vi "SubPanelBasicFlow.vi"(0 "VI Reference In":refnum<vi>, 1 "Label (VI Title)":string="Default", 11 "error in (no error)":errorcluster) -> (4 "VI Reference Out":refnum<vi>, 15 "error out":errorcluster)   [LabVIEW 2016, in "Drona Test.lvlib"]
uses:
  Drona Test.lvlib
  main/apis/Stimulus/ValueSignal/ValueSignalByPathString.vi
  main/apis/Assert/AssertControlValue/Equal.vi
  <vilib>/addons/_JKI Toolkits/Caraya/classes/Assert/Assert Not Error.vi
  <vilib>/addons/_JKI Toolkits/Caraya/classes/Test/Test.lvclass
  main/Drona.lvlib
  <vilib>/addons/_JKI Toolkits/Caraya/classes/Assert/Assert.lvclass
  main/apis/Assert/AssertControlValue/AssertControlValue.lvlib
  main/apis/Stimulus/ValueSignal/ValueSignal.lvlib
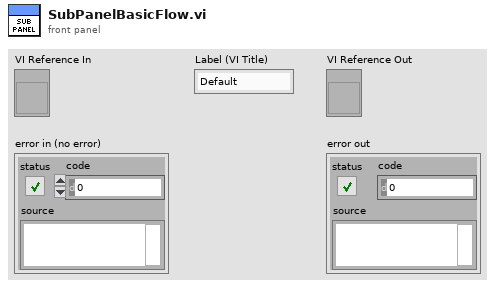
[diagram p1: front panel]
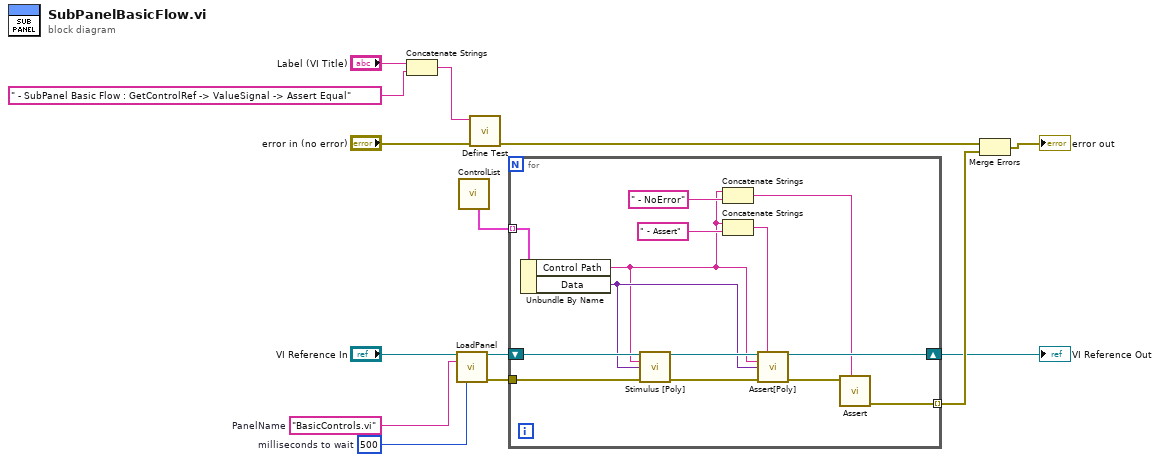
[diagram p0: block diagram]
diagram:
  w4 = u32 500  # milliseconds to wait
  w5 = "BasicControls.vi"  # PanelName
  n1 = Concatenate Strings("Label (VI Title)", " - SubPanel Basic Flow : GetControlRef -> ValueSignal -> Assert Equal" ("Label (VI Title)")) -> (w7:string)
  n2 = call "LoadPanel.vi"("VI in"="VI Reference In", "Panel Name"=w5, "milliseconds to wait"=w4) -> ("VI out"=w2:refnum<vi>, "error out"=w1:errorcluster)  [unwired: 11 in]
  n3 = call "ControlList.vi"() -> ("SubPanel"=w6:cluster{"Control Path":string, "Data":variant}[])  [unwired: 6 in, 5 out]
  n4 = call <vilib>:"Define Test.vi"("error in (no error)"="error in (no error)", "Label (VI Title)"=w7) -> ("error out"=w10:errorcluster)  [unwired: 9 in]
  n5 = for {
    shift-right: [w28] -> w12
    shift-left: w2 -> [w24]
    tunnel: [w16] -> w14 mode=indexing
    tunnel: w6 -> [w25] mode=indexing
    tunnel: w1 -> [w15]
    n6 = Unbundle By Name(w25) -> ("Control Path"=w19:string, "Data"=w23:variant)
    n7 = call-poly "Stimulus [Poly].vi"("VI Reference In"=w24, "Control Path"=w19, "Value (Signaling)"=w23, "error in"=w15) -> ("VI Reference Out"=w26:refnum<vi>, "error out"=w27:errorcluster)  [unwired: 10 in]
    n8 = Concatenate Strings(w19, " - NoError" ("string")) -> (w17:string)
    n9 = Concatenate Strings(w19, " - Assert" ("string")) -> (w21:string)
    n10 = call-poly "Assert[Poly].vi"("VI Reference In"=w26, "Label"=w21, "Control Path"=w19, "Control Value"=w23, "Error In"=w27) -> ("VI Reference Out"=w28:refnum<vi>, "Error Out"=w18:errorcluster)  [unwired: 9 in]
    n11 = call-poly <vilib>:"Assert.vi"("Label"=w17, "Not Error?"=w18) -> ("error out"=w16:errorcluster)  [unwired: 9 in]
  }
  "VI Reference Out" <- w12
  n12 = Merge Errors(w10, w14) -> (→"error out":errorcluster)
